vi "标定授权读取.vi"(1 "VCI_Receive":T1 {"Rsv3" max=0 format="%x"; "Rsv2" min=101 format="%x"; "Rsv1" format="%x"; "Data8" format="%x"; "Data7" format="%x"; "Data6" format="%x"; "Data5" format="%x"; "Data4" format="%x"; "Data3" format="%x"; "Data2" format="%x"; "Data1" format="%x"; "DataLen" format="%x"; "ExternFlag" format="%x"; "RemoteFlag" format="%x"; "SendType" format="%x"; "TimeFlag" format="%x"; "TimeStamp" format="%x"; "ID" format="%x"}) -> ()   [LabVIEW 2013]
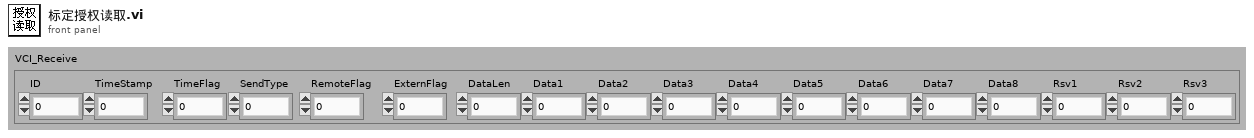
[diagram p1: front panel]
types:
  T1 = cluster{"ID":u32, "TimeStamp":u32, "TimeFlag":u8, "SendType":u8, "RemoteFlag":u8, "ExternFlag":u8, "DataLen":u8, "Data1":u8, "Data2":u8, "Data3":u8, "Data4":u8, "Data5":u8, "Data6":u8, "Data7":u8, "Data8":u8, "Rsv1":u8, "Rsv2":u8, "Rsv3":u8}
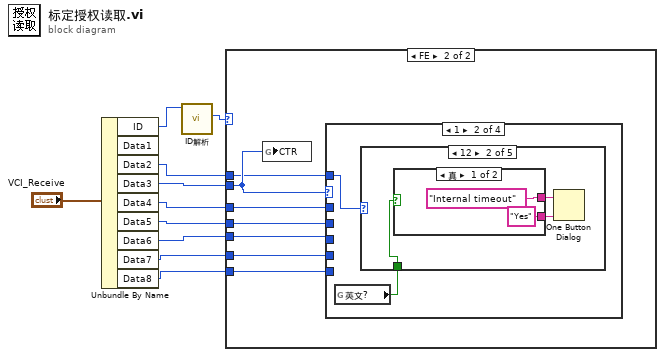
[diagram p0: block diagram]
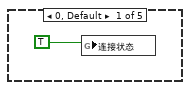
[diagram p4: hidden frame]
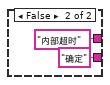
[diagram p5: hidden frame]
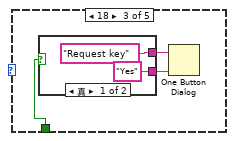
[diagram p6: hidden frame]
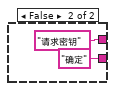
[diagram p7: hidden frame]
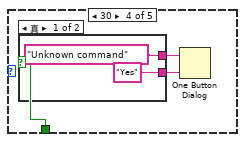
[diagram p8: hidden frame]
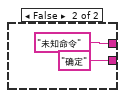
[diagram p9: hidden frame]
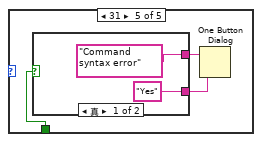
[diagram p10: hidden frame]
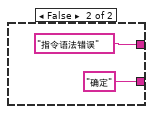
[diagram p11: hidden frame]
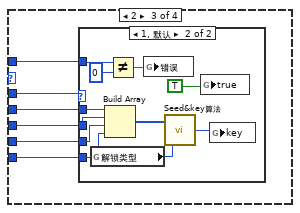
[diagram p12: hidden frame]
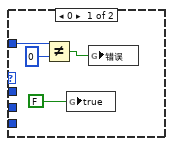
[diagram p13: hidden frame]
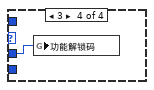
[diagram p14: hidden frame]
diagram:
  n1 = Unbundle By Name("VCI_Receive") -> ("ID"=w3:u32, "Data2"=w4:u8, "Data3"=w5:u8, "Data4"=w6:u8, "Data5"=w7:u8, "Data6"=w8:u8, "Data7"=w9:u8, "Data8"=w10:u8)  [unwired: 1 out]
  n2 = call "ID解析.vi"("ID"=w3) -> ("PF(2)"=w2:i32)  [unwired: 10 out]
  n3 = case shown="FE" w2 {
    tunnel: w10 -> [_ w17]
    tunnel: w9 -> [_ w16]
    tunnel: w8 -> [_ w15]
    tunnel: w7 -> [_ w14]
    tunnel: w6 -> [_ w13]
    tunnel: w5 -> [_ w12]
    tunnel: w4 -> [_ w11]
    frame 0, Default {
    }
    frame 254 {
      n4 = global write "标定授权全局.vi" "CTR"(w12) -> ()
      n5 = case shown="1" w12 {
        tunnel: w11 -> [_ w19 w49 _]
        tunnel: w17 -> [_ _ w51 _]
        tunnel: w16 -> [_ _ w52 _]
        tunnel: w15 -> [_ _ w53 _]
        tunnel: w14 -> [_ _ w54 _]
        tunnel: w13 -> [_ _ w50 w70]
        frame 0, Default {
        }
        frame 1 {
          n6 = global read "中英文全局-8.6.vi" "英文?"() -> (w18:bool)
          n7 = case shown="12" w19 {
            tunnel: w18 -> [_ w21 w28 w35 w42]
            frame 0, Default {
              n8 = global write "标定授权全局.vi" "连接状态"(TRUE ("true")) -> ()
            }
            frame 12 {
              n9 = case shown="真" w21 {
                tunnel: ["Internal timeout" ("消息") "内部超时" ("消息")] -> w23
                tunnel: ["Yes" ("按钮名称（“确定”）") "确定" ("按钮名称（“确定”）")] -> w22
                frame True {
                }
                frame False {
                }
              }
              n10 = One Button Dialog(message=w23, button name ("OK")=w22) -> ()  [unwired: 1 out]
            }
            frame 18 {
              n11 = case shown="真" w28 {
                tunnel: ["Request key" ("消息") "请求密钥" ("消息")] -> w30
                tunnel: ["Yes" ("按钮名称（“确定”）") "确定" ("按钮名称（“确定”）")] -> w29
                frame True {
                }
                frame False {
                }
              }
              n12 = One Button Dialog(message=w30, button name ("OK")=w29) -> ()  [unwired: 1 out]
            }
            frame 30 {
              n13 = case shown="真" w35 {
                tunnel: ["Unknown command" ("消息") "未知命令" ("消息")] -> w37
                tunnel: ["Yes" ("按钮名称（“确定”）") "确定" ("按钮名称（“确定”）")] -> w36
                frame True {
                }
                frame False {
                }
              }
              n14 = One Button Dialog(message=w37, button name ("OK")=w36) -> ()  [unwired: 1 out]
            }
            frame 31 {
              n15 = case shown="真" w42 {
                tunnel: ["Command syntax error" ("消息") "指令语法错误" ("消息")] -> w44
                tunnel: ["Yes" ("按钮名称（“确定”）") "确定" ("按钮名称（“确定”）")] -> w43
                frame True {
                }
                frame False {
                }
              }
              n16 = One Button Dialog(message=w44, button name ("OK")=w43) -> ()  [unwired: 1 out]
            }
          }
        }
        frame 2 {
          n17 = case shown="1, 默认" w50 {
            tunnel: w54 -> [_ w69]
            tunnel: w53 -> [_ w68]
            tunnel: w52 -> [_ w67]
            tunnel: w51 -> [_ w66]
            tunnel: w49 -> [w57 w64]
            frame 0 {
              n18 = Not Equal?(x=w57, y=u8 0) -> (x != y?=w55:bool)
              n19 = global write "标定授权全局.vi" "true"(FALSE ("true")) -> ()
              n20 = global write "标定授权全局.vi" "错误"(w55) -> ()
            }
            frame 1, Default {
              n21 = global read "标定授权全局.vi" "解锁类型"() -> (w59:enum16{"读取", "写", "下载"})
              n22 = Build Array(w69, w68, w67, w66) -> (w65:u8[])
              n23 = Not Equal?(x=w64, y=u8 0) -> (x != y?=w62:bool)
              n24 = global write "标定授权全局.vi" "错误"(w62) -> ()
              n25 = call "Seed&key算法.vi"("解锁类型"=w59, "Seed"=w65) -> ("key"=w60:u32)
              n26 = global write "标定授权全局.vi" "true"(TRUE ("true")) -> ()
              n27 = global write "标定授权全局.vi" "key"(w60) -> ()
            }
          }
        }
        frame 3 {
          n28 = global write "标定授权全局.vi" "功能解锁码"(w70) -> ()
        }
      }
    }
  }
